vi "CoilsSet.vi"(7 "Settings":cluster{"x":dbl, "y":dbl, "z":dbl, "axgrad":dbl}, 8 "error in":errorcluster, 9 "DO Task":refnum<k21>, 10 "AO Task":refnum<k21>, 11 "Keithley USB":refnum<visa-resource-name>) -> (0 "error out":errorcluster, 1 "DO Task out":refnum<k21>, 2 "AO Task out":refnum<k21>, 3 "Keithley USB out":refnum<visa-resource-name>)   [LabVIEW 2012]
uses:
  <vilib>/DAQmx/write.llb/DAQmx Write (Analog DBL 1Chan 1Samp).vi
  <vilib>/DAQmx/write.llb/DAQmx Write (Digital 1D Bool 1Chan 1Samp).vi
  <vilib>/DAQmx/miscellaneous.llb/DAQmx Fill In Error Info.vi
panel:
  # "(A)"
  # "(A)"
  # "(A)"
  # "(DAC V)"
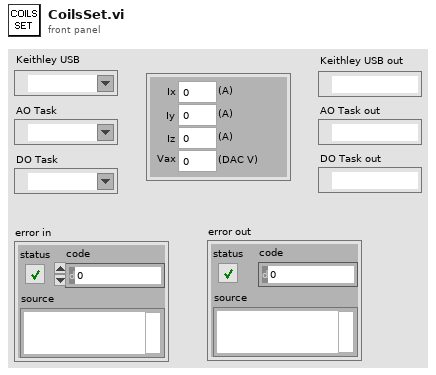
[diagram p1: front panel]
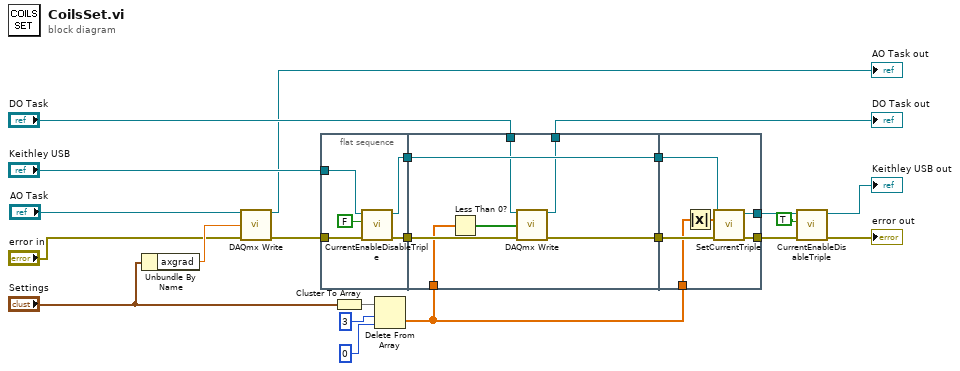
[diagram p0: block diagram]
diagram:
  n1 = Unbundle By Name("Settings") -> ("axgrad"=w14:dbl)
  n2 = call-poly <vilib>:"DAQmx Write.vi"("task/channels in"="AO Task", "data"=w14, "error in"="error in") -> ("task out"=→"AO Task out":refnum<k21>, "error out"=w1:errorcluster)  [unwired: 10 in, 1 out]
  n3 = flat-sequence {
    tunnel: [w26] -> w9
    tunnel: [w25] -> w8
    tunnel: "Keithley USB" -> [w24]
    tunnel: w1 -> [w23]
    tunnel: [w31] -> w7
    tunnel: w9 -> [w32]
    tunnel: [w34] -> w6
    tunnel: w8 -> [w34]
    tunnel: "DO Task" -> [w33]
    tunnel: [w30] -> w15
    tunnel: w2 -> [w29]
    tunnel: [w40] -> w5
    tunnel: [w39] -> w4
    tunnel: w7 -> [w38]
    tunnel: w6 -> [w37]
    tunnel: w2 -> [w35]
    frame #0 {
      n4 = call "CurrentEnableDisableTriple.vi"("error in (no error)"=w23, "Enable Output (T: On)"=FALSE, "Visa Resource Name In"=w24) -> ("error in (no error) 2"=w26:errorcluster, "Visa Resource Name Out"=w25:refnum<visa-resource-name>)  [unwired: 7 in]
    }
    frame #1 {
      n5 = Less Than 0?(x=w29) -> (x < 0?=w28:bool[])
      n6 = call-poly <vilib>:"DAQmx Write.vi"("task/channels in"=w33, "data"=w28, "error in"=w32) -> ("task out"=w30:refnum<k21>, "error out"=w31:errorcluster)  [unwired: 10 in, 1 out]
    }
    frame #2 {
      n7 = Absolute Value(x=w35) -> (abs(x)=w36:dbl[])
      n8 = call "SetCurrentTriple.vi"("error in"=w38, "Current"=w36, "VISA resource name in"=w37) -> ("error out"=w40:errorcluster, "VISA resource name out"=w39:refnum<visa-resource-name>)  [unwired: 7 in]
    }
  }
  n9 = Cluster To Array(cluster="Settings") -> (array=w11:dbl[])
  n10 = Delete From Array(array=w11, length=3, index=0) -> (deleted portion=w2:dbl[])  [unwired: 1 out]
  n11 = call "CurrentEnableDisableTriple.vi"("error in (no error)"=w5, "Enable Output (T: On)"=TRUE, "Visa Resource Name In"=w4) -> ("error in (no error) 2"=→"error out":errorcluster, "Visa Resource Name Out"=→"Keithley USB out":refnum<visa-resource-name>)  [unwired: 7 in]
  "DO Task out" <- w15
